vi "SPI Engine.SPICore.InputBuffer.vi"(6 "Ready for Output":bool, 9 "Input Valid":bool, 10 "SPI Information In":T1) -> (1 "Output Data":bool, 2 "SPI Information Out":T1, 4 "Ready For Input":bool)   [LabVIEW 2014]
uses:
  Controls/SPI Transaction Packet.ctl
  <vilib>/rvi/Emulation/niFpgaSctlEmulationGetInTimedLoop.vi
  <vilib>/rvi/DataTransferAndStorage/Container/Common/niFpgaContainerGetUniqueNameForEmu.vi
  <vilib>/rvi/DataTransferAndStorage/Container/Common/niFpgaContainerSetEmuInfo.vi
  <vilib>/rvi/eio/common/nirviEmuReportErrorAndStop.vi
  <vilib>/rvi/DataTransferAndStorage/Container/Common/niFpgaContainerExecOnDevCompGetState.vi
  <vilib>/rvi/Emulation/niFpgaEmulationIsFPGAContextNoSignature.vi
  <vilib>/rvi/errors/niFpgaSetErrorForExecOnDevCompSimple.vi
  <vilib>/rvi/FIFO/Fifo_Resource/nirvififoEmulationSetSize.vi
  <vilib>/rvi/FIFO/Fifo_Resource/nirviFifoEmulationQueueMgr.vi
  <instcachedir>/0/nirviFifoEmulationQueueMgr_E5CAEC123FF24DC58D834DCA3CDAA9B5.lvgen/nirviFifoEmulationQueueMgr_E5CAEC123FF24DC58D834DCA3CDAA9B5_003.vi
  <vilib>/rvi/FIFO/Fifo_Resource/nirvififoEmulationDetermineInputValidOut.vi
  <vilib>/rvi/FIFO/Fifo_Resource/nirvififoEmulationCreateLock.vi
  <vilib>/rvi/Emulation/niFpgaProcessEmulError.vi
  <vilib>/rvi/FIFO/Fifo_Resource/nirvififoEmulationObtainLock.vi
  <vilib>/rvi/FIFO/Fifo_Resource/nirvififoEmulationReleaseLock.vi
  <vilib>/rvi/occurrence/nirviWaitOnOccurrenceBase.vi
  <vilib>/rvi/errors/nirviReportUnexpectedCaseInternalError.vi
  <vilib>/rvi/errors/nirviReportUnexpectedCaseInternalError (U32).vi
  <vilib>/rvi/interface/RandomDataEmulation/niFpgaRandomDataHandleErrors.vi
  <vilib>/rvi/LocalResourceManager/LocalResourceManager.xnode
  <vilib>/rvi/DataTransferAndStorage/Container/XNode/niFpgaContainer.xnode
  <vilib>/rvi/FIFO/Fifo_Resource/niFpgaFifoEmulationRefIn.vi
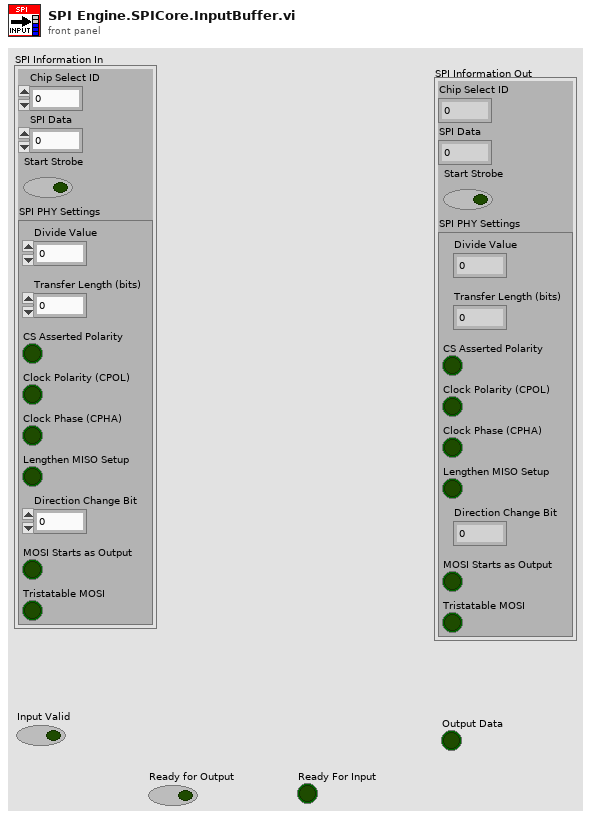
[diagram p1: front panel]
types:
  T1 = typedef "SPI Transaction Packet.ctl" = cluster{"Chip Select ID":u8, "SPI Data":u64, "Start Strobe":bool, "SPI PHY Settings":cluster{"Divide Value":u8, "Transfer Length (bits)":u8, "CS Asserted Polarity":bool, "Clock Polarity (CPOL)":bool, "Clock Phase (CPHA)":bool, "Lengthen MISO Setup":bool, "Direction Change Bit":u8, "MOSI Starts as Output":bool, "Tristatable MOSI":bool}}
  T2 = cluster{"Chip Select ID":u8, "SPI Data":u64, "Start Strobe":bool, "SPI PHY Settings":cluster{"Divide Value":u8, "Transfer Length (bits)":u8, "CS Asserted Polarity":bool, "Clock Polarity (CPOL)":bool, "Clock Phase (CPHA)":bool, "Lengthen MISO Setup":bool, "Direction Change Bit":u8, "MOSI Starts as Output":bool, "Tristatable MOSI":bool}}
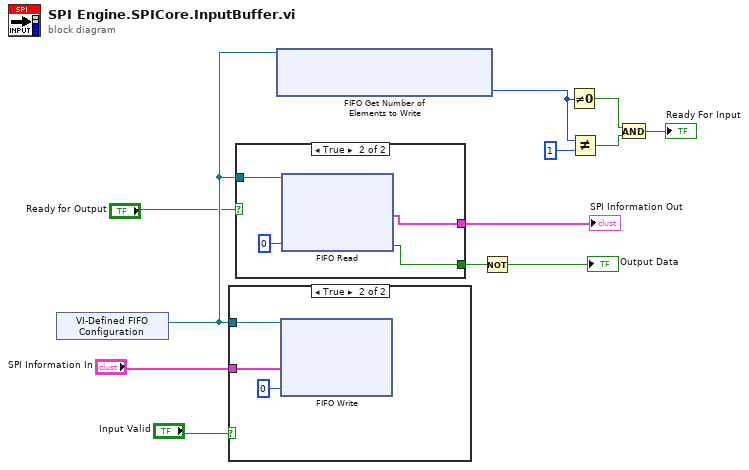
[diagram p0: block diagram]
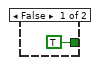
[diagram p2: hidden frame]
diagram:
  n1 = xnode "VI-Defined FIFO Configuration"() -> ("FIFO Out"=w10:refnum<k21>)
  n2 = case shown="True" "Input Valid" {
    tunnel: "SPI Information In" -> [_ w15]
    tunnel: w10 -> [_ w13]
    frame False {
    }
    frame True {
      n3 = xnode "FIFO Write"("Element"=w15, "Timeout"=0, "FIFO In"=w13) -> ()  [unwired: 2 out]
    }
  }
  n4 = case shown="True" "Ready for Output" {
    tunnel: [_ w19] -> w1
    tunnel: [TRUE ("Timed Out?") w18] -> w12
    tunnel: w10 -> [_ w17]
    frame False {
    }
    frame True {
      n5 = xnode "FIFO Read"("Timeout"=0, "FIFO In"=w17) -> ("Element"=w19:T2, "Timed Out?"=w18:bool)  [unwired: 1 out]
    }
  }
  "SPI Information Out" <- w1
  n6 = xnode "FIFO Get Number of Elements to Write"("FIFO In"=w10) -> ("Number of Elements to Write"=w9:u32)  [unwired: 1 out]
  n7 = Not(x=w12) -> (.not. x?=→"Output Data":bool)
  n8 = Not Equal To 0?(x=w9) -> (x != 0?=w7:bool)
  n9 = Not Equal?(x=w9, y=u32 1) -> (x != y?=w8:bool)
  n10 = And(x=w7, y=w8) -> (x .and. y?=→"Ready For Input":bool)
